vi "picoscopeMemoryAllocationAndAcquisition.vi"(8 "error in (no error)":errorcluster, 11 "PicoscopeV2 in":refnum<class "PicoscopeV2.lvclass">) -> (0 "error out":errorcluster, 1 "Properties Panel 2":T2, 2 "handle out":i16, 3 "Data Pointers":T3, 5 "Segment Range":T1 {"toSegmentIndex" format="%.4p"; "fromSegmentIndex" format="%.4p"})   [LabVIEW 2020, in "PicoscopeV2.lvclass"]
uses:
  PicoscopeV2.lvclass
  PicoBuffers.ctl
  Segment Range.ctl
  PicoscopeV2.lvclass/PicoscopeV2.ctl
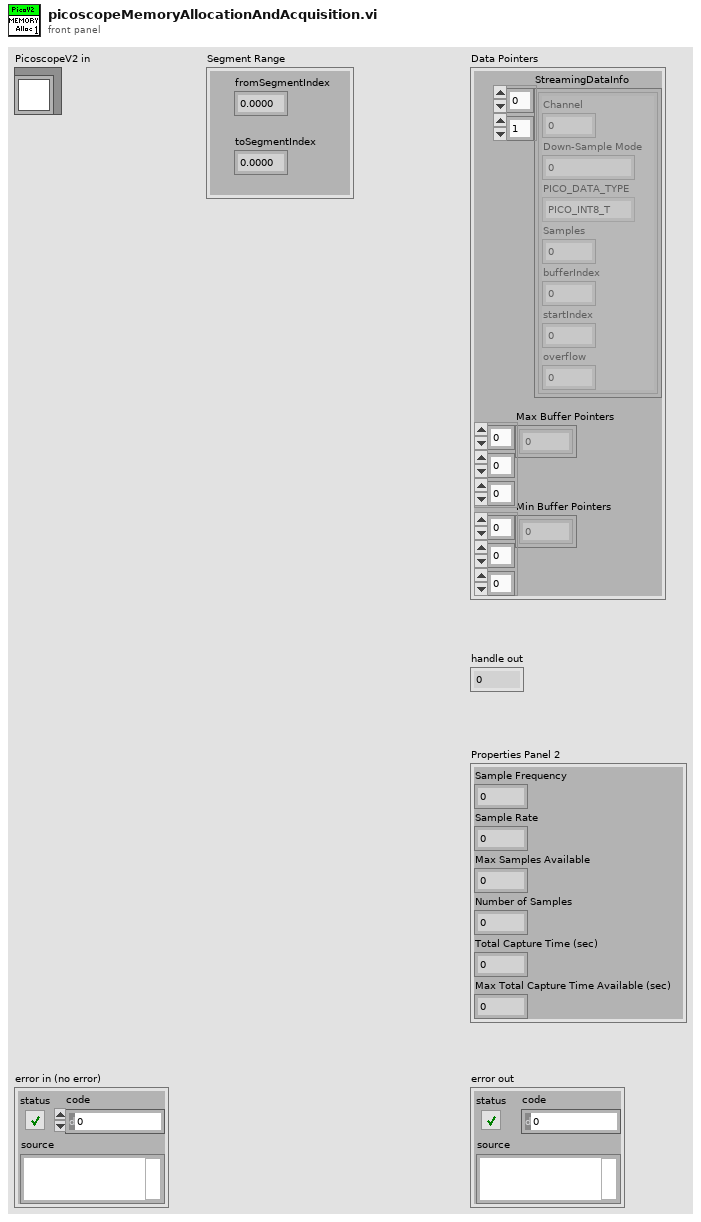
[diagram p1: front panel]
types:
  T1 = typedef "Segment Range.ctl" = cluster{"fromSegmentIndex":u64, "toSegmentIndex":u64}
  T2 = cluster{"Sample Frequency":sgl, "Sample Rate":sgl, "Max Samples Available":i32, "Number of Samples":u32, "Total Capture Time (sec) ":sgl, "Max Total Capture Time Available (sec)":sgl}
  T3 = typedef "PicoBuffers.ctl" = cluster{"Max Buffer Pointers":u64[][][], "Min Buffer Pointers":u64[][][], "StreamingDataInfo":cluster{"Channel":u32, "Down-Sample Mode":u32, "PICO_DATA_TYPE":enum32{"PICO_INT8_T", "PICO_INT16_T", "PICO_INT32_T", "PICO_UINT32_T", "PICO_INT64_T", ""}, "Samples":i32, "bufferIndex":u64, "startIndex":i32, "overflow":i16}[][]}
  T4 = typedef "Acquisition Settings.ctl" = cluster{"preTriggerSamples":u64, "postTriggerSamples":u64, "timebase":u32}
  T5 = typedef "Buffer and Transfer Settings.ctl" = cluster{"startIndex":u64, "Samples":u64, "Down Sample Ratio":u64, "Down-Sample Mode":u32}
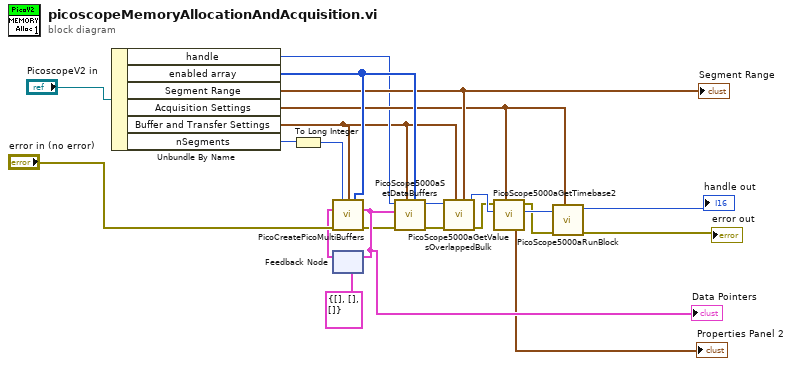
[diagram p0: block diagram]
diagram:
  n1 = Unbundle By Name("PicoscopeV2 in") -> ("handle"=w8:i16, "enabled array"=w20:i16[], "Segment Range"=w16:T1, "Acquisition Settings"=w15:T4, "Buffer and Transfer Settings"=w2:T5, "nSegments"=w1:i32)
  "Segment Range" <- w16
  n2 = To Long Integer(number=w1) -> (32bit integer=w5:i32)
  n3 = feedback #1(T3 {"Max Buffer Pointers"=[], "Min Buffer Pointers"=[], "StreamingDataInfo"=[]} ("Data Pointers")) -> (w4:T3)
  n4 = call "PicoCreatePicoMultiBuffers.vi"("Number of Buffers"=w5, "Buffer and Transfer Settings"=w2, "enabled array"=w20, "Data Pointers In"=w4, "error in (no error)"="error in (no error)") -> ("Data Pointers"=w18:T3, "error out"=w7:errorcluster)  [unwired: 9 in]
  "Data Pointers" <- w18
  n5 = feedback-in #1(w18) -> ()
  n6 = call "PicoScope5000aSetDataBuffers.vi"("enabled array"=w20, "Buffer and Transfer Settings"=w2, "error in (no error)"=w7, "Data Pointers In"=w18, "handle in"=w8) -> ("error out"=w9:errorcluster, "handle out"=w10:i16)  [unwired: 5 in]
  n7 = call "PicoScope5000aGetValuesOverlappedBulk.vi"("Segment Range"=w16, "Buffer and Transfer Settings"=w2, "error in (no error)"=w9, "handle in"=w10) -> ("error out"=w11:errorcluster, "handle out"=w12:i16)  [unwired: 4 in, 2 out]
  n8 = call "PicoScope5000aGetTimebase2.vi"("Acquisition Settings"=w15, "handle in"=w12, "error in (no error)"=w11) -> ("handle out"=w14:i16, "error out"=w13:errorcluster, "Properties Panel"=→"Properties Panel 2":T2)  [unwired: 6 in]
  n9 = call "PicoScope5000aRunBlock.vi"("Acquisition Settings"=w15, "error in (no error)"=w13, "handle in"=w14) -> ("error out"=→"error out":errorcluster, "handle out"=→"handle out":i16)  [unwired: 5 in, 2 out]
